vi "GainDB.vi"(1 "Vin":ext, 2 "Vout":ext) -> (0 "Gain dB":ext)   [LabVIEW 2014]
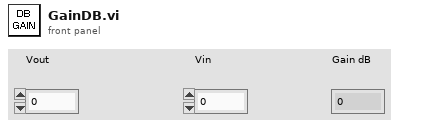
[diagram p1: front panel]
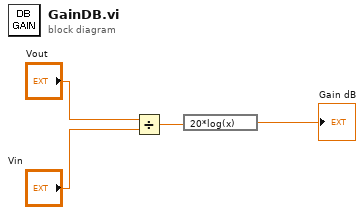
[diagram p0: block diagram]
diagram:
  n1 = Divide(x="Vout", y="Vin") -> (x/y=w2:ext)
  n2 = expression code="20*log(x)"(w2) -> (→"Gain dB":ext)
